vi "Read configuration.vi"(8 "error in":errorcluster, 11 "ThreePhasePLL editor node in":refnum<class "ThreePhasePLL editor node.lvclass">) -> (0 "error out":errorcluster, 2 "configuration":refnum<class "NISE_CEF_serializable configuration.lvclass">, 3 "ThreePhasePLL editor node out":refnum<class "ThreePhasePLL editor node.lvclass">)   [LabVIEW 2017, in "ThreePhasePLL editor node.lvclass"]
uses:
  ThreePhasePLL editor node.lvclass
  <vilib>/NI/Configuration Framework/serializable configuration/NISE_CEF_serializable configuration.lvclass
  ThreePhasePLL editor node.lvclass/ThreePhasePLL editor node.ctl
  module/configuration/ThreePhasePLL configuration.lvclass
  C:/Program Files (x86)/National Instruments/LabVIEW 2017/vi.lib/NI/Configuration Framework/serializable configuration/NISE_CEF_serializable configuration.lvclass
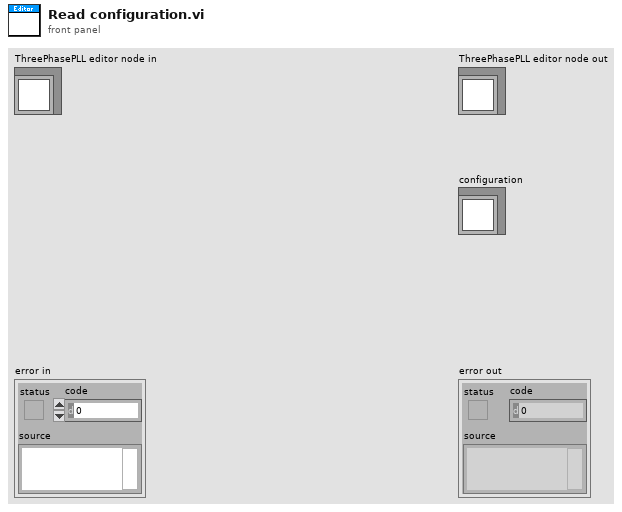
[diagram p1: front panel]
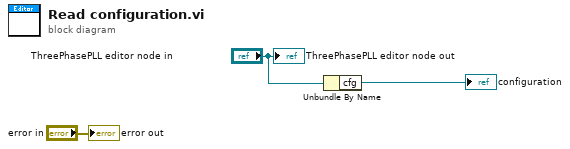
[diagram p0: block diagram]
diagram:
  n1 = Unbundle By Name("ThreePhasePLL editor node in") -> ("cfg"=→"configuration":refnum<class "ThreePhasePLL configuration.lvclass">)
  "error out" <- "error in"
  "ThreePhasePLL editor node out" <- "ThreePhasePLL editor node in"
